vi "Autonomous Independent.vi"() -> ()   [LabVIEW 2016]
doc: "This VI is called when autonomous begins, and will automatically be terminated when autonomous ends. You can carry out timed or sensor driven robot movement independently without needing to return to the caller."
uses:
  <vilib>/Rock Robotics/WPI/Utilities/WPI_GetSetVariantRefNum.vi
  <vilib>/Rock Robotics/Network Tables/NT Write Numeric Array.vi
  Robot Global Data.vi
  <vilib>/Rock Robotics/WPI/RobotDrive/WPI_RobotDriveArcadeDrive_Standard(NoSaturation).vi
panel:
  in  "Drive to target":bool=TRUE
  in  "Auto Routine":enum16{"PID Angle Testing", "Find Target"}(ring)=enum."Find Target"
  # "Be sure to right-click and choose Data Operations>>Make Current Value default if you want to save the array values with the VI"
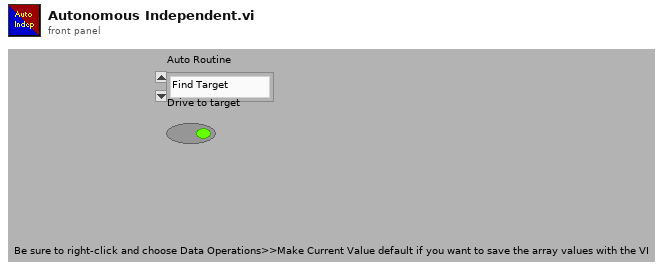
[diagram p1: front panel]
types:
  T1 = typedef "WPI_JoystickDevRef.ctl" = cluster{"Device":T2}
  T2 = typedef "WPI_JoystickDeviceEnum.ctl" = enum16{"USB 0", "USB 1", "USB 2", "USB 3", "USB 4", "USB 5"}
  T3 = typedef "WPI_RobotDriveDevRef.ctl" = cluster{"DevStatus":errorcluster, "Motors[]":T4[], "Square Inputs":bool, "Max Output":dbl}
  T4 = typedef "WPI_MotorControlDeviceRef.ctl" = cluster{"DeviceStatus":errorcluster, "Type":T5, "PWM":cluster{"PWM Channel":T6, "DeadBand":T7}, "CAN":cluster{"Device Number":u8, "SetOutput VI Ref":variant, "GetOutput VI Ref":variant, "Enable VI Ref":variant, "Disable VI Ref":variant, "Data":variant}, "Invert":bool}
  T5 = typedef "WPI_MotorControlType.ctl" = enum16{"PWM", "CAN"}
  T6 = typedef "FPGA_DIOPWMChannel.ctl" = enum8{"PWM 0", "PWM 1", "PWM 2", "PWM 3", "PWM 4", "PWM 5", "PWM 6", "PWM 7", "PWM 8", "PWM 9", "PWM MXP 0", "PWM MXP 1", "PWM MXP 2", "PWM MXP 3", "PWM MXP 4", "PWM MXP 5", "PWM MXP 6", "PWM MXP 7", "PWM MXP 8", "PWM MXP 9", "Invalid"}
  T7 = typedef "WPI_PWMDeadband.ctl" = cluster{"Name":string, "maxPositivePwm":i32, "minPositivePwm":i32, "centerPwm":i32, "maxNegativePwm":i32, "minNegativePwm":i32, "angularRange":u16}
  T8 = cluster{"Target?":bool, "Angle":dbl, "Distance":dbl}
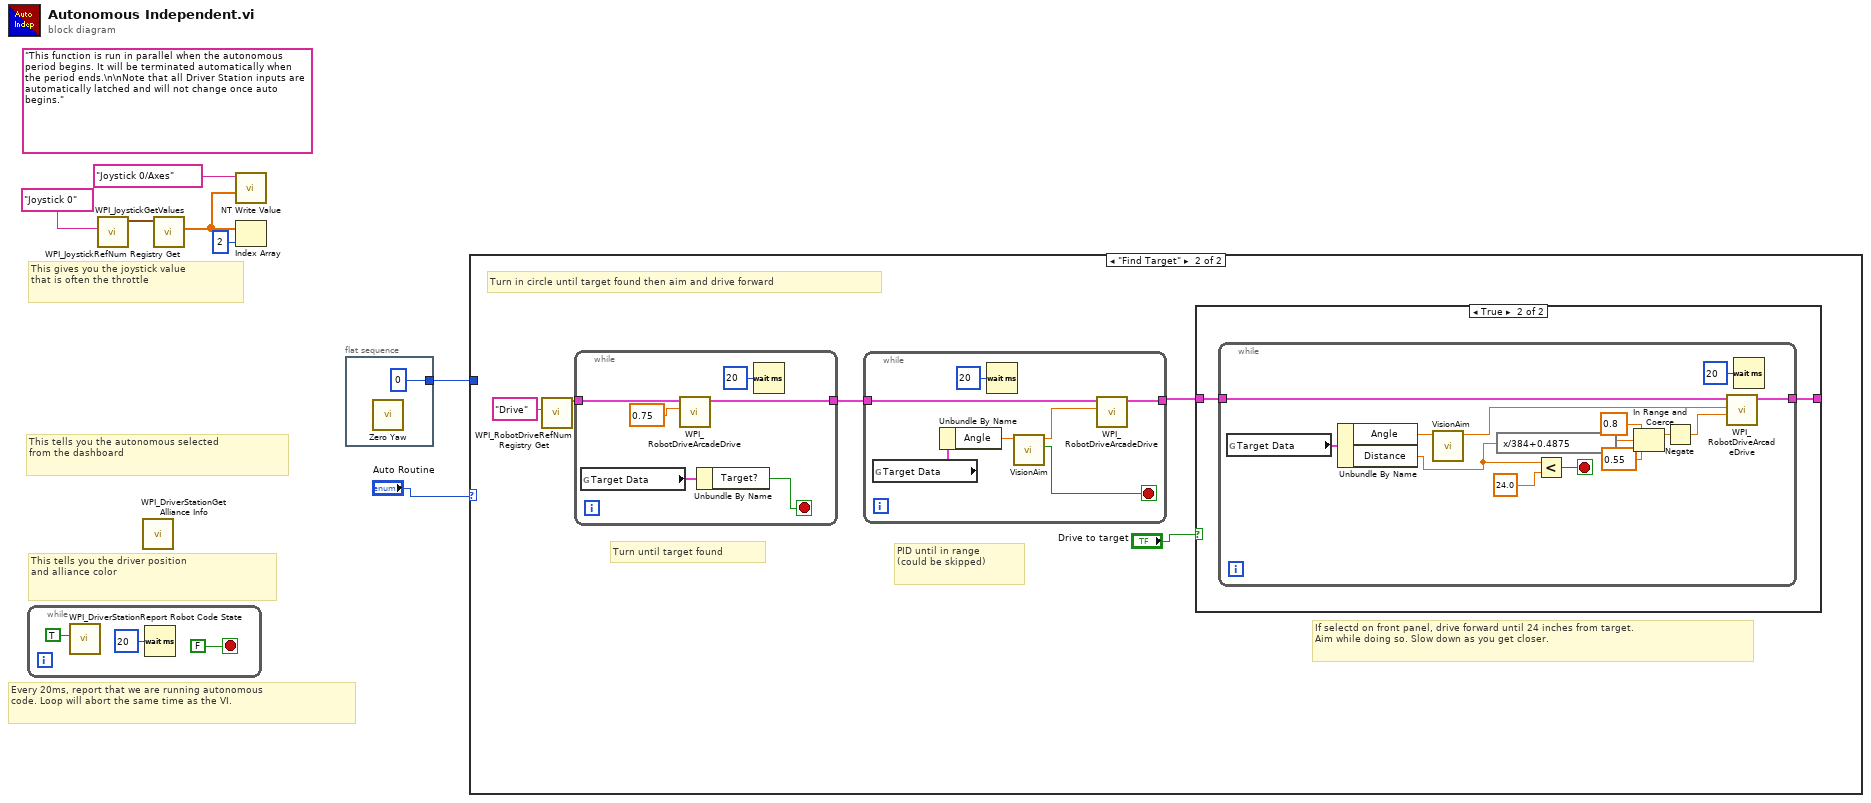
[diagram p0: block diagram]
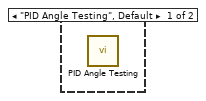
[diagram p2: hidden frame]
diagram:
  (unwired) "This function is run in parallel when the autonomous period begins. It will be terminated automatically when the period ends.\n\nNote that all Driver Station inputs are automatically latched and will not change once auto begins."
  # "This tells you the autonomous selected\nfrom the dashboard"
  # "Every 20ms, report that we are running autonomous\ncode. Loop will abort the same time as the VI."
  # "This gives you the joystick value\nthat is often the throttle"
  # "This tells you the driver position\nand alliance color"
  n1 = while {
    stop <- FALSE stop-if-true
    n2 = call <vilib>:"WPI_DriverStationReport Robot Code State.vi"("Autonomous"=TRUE) -> ()  [unwired: 10 in, 1 out]
    n3 = Wait (ms)(milliseconds to wait=u32 20) -> ()  [unwired: 1 out]
  }
  n4 = call <vilib>:"WPI_JoystickRefNum Registry Get.vi"("refnum name"="Joystick 0") -> ("JoystickDevRef"=w6:T1)  [unwired: 1 in, 9 out]
  n5 = call <vilib>:"WPI_DriverStationGet Alliance Info.vi"() -> ()  [unwired: 12 out]
  n6 = call <vilib>:"WPI_JoystickGetValues.vi"("JoystickDevRef"=w6) -> ("Axes"=w4:dbl[])  [unwired: 6 in, 4 out]
  n7 = call-poly <vilib>:"NT Write Value.vi"("Numeric Array"=w4, "Name"="Joystick 0/Axes") -> ()  [unwired: 9 in, 1 out]
  n8 = Index Array(array=w4, index=2) -> ()  [unwired: 1 out]
  n9 = flat-sequence {
    tunnel: [u32 0 ("milliseconds to wait")] -> w1
    frame #0 {
      n10 = call <vilib>:"Zero Yaw.vi"() -> ()  [unwired: 12 in]
    }
  }
  n11 = case shown="\"Find Target\"" "Auto Routine" {
    tunnel: w1 -> [_ _]
    frame "PID Angle Testing", Default {
      n12 = call "PID Angle Testing.vi"() -> ()  [unwired: 12 in]
    }
    frame "Find Target" {
      # "If selectd on front panel, drive forward until 24 inches from target.\nAim while doing so. Slow down as you get closer."
      # "PID until in range\n(could be skipped)"
      # "Turn until target found"
      # "Turn in circle until target found then aim and drive forward"
      n13 = call <vilib>:"WPI_RobotDriveRefNum Registry Get.vi"("refnum name"="Drive") -> ("RobotDriveDevRef"=w15:T3)  [unwired: 9 in, 1 out]
      n14 = while {
        tunnel: w15 -> [w46]
        tunnel: [w44] -> w14
        stop <- w41 stop-if-true
        n15 = global read "Robot Global Data.vi" "Target Data"() -> (w42:T8)
        n16 = call-poly <vilib>:"WPI_RobotDriveArcadeDrive.vi"("X axis value"=0.75, "RobotDriveDevRef"=w46) -> ("RobotDriveDevRef"=w44:T3)  [unwired: 7 in, 2 out]
        n17 = Unbundle By Name(w42) -> ("Target?"=w41:bool)
        n18 = Wait (ms)(milliseconds to wait=u32 20) -> ()  [unwired: 1 out]
      }
      n19 = while {
        tunnel: w14 -> [w40]
        tunnel: [w36] -> w12
        stop <- w38 stop-if-true
        n20 = global read "Robot Global Data.vi" "Target Data"() -> (w35:T8)
        n21 = Unbundle By Name(w35) -> ("Angle"=w34:dbl)
        n22 = Wait (ms)(milliseconds to wait=u32 20) -> ()  [unwired: 1 out]
        n23 = call "VisionAim.vi"("Angle"=w34) -> ("In Range"=w38:bool, "Turn Amount"=w39:dbl)  [unwired: 9 in]
        n24 = call-poly <vilib>:"WPI_RobotDriveArcadeDrive.vi"("X axis value"=w39, "RobotDriveDevRef"=w40) -> ("RobotDriveDevRef"=w36:T3)  [unwired: 7 in, 2 out]
      }
      n25 = case shown="True" "Drive to target" {
        tunnel: w12 -> [w17 w19]
        tunnel: [w17 w18] -> _
        frame False {
        }
        frame True {
          n26 = while {
            tunnel: w19 -> [w32]
            tunnel: [w31] -> w18
            stop <- w29 stop-if-true
            n27 = global read "Robot Global Data.vi" "Target Data"() -> (w22:T8)
            n28 = Unbundle By Name(w22) -> ("Angle"=w21:dbl, "Distance"=w20:dbl)
            n29 = call "VisionAim.vi"("Angle"=w21) -> ("Turn Amount"=w33:dbl)  [unwired: 9 in, 1 out]
            n30 = expression code="x/384+0.4875"(w20) -> (w27:dbl)
            n31 = Less?(x=w20, y=24.0) -> (x < y?=w29:bool)
            n32 = In Range and Coerce(upper limit=0.8, x=w27, lower limit=0.55) -> (coerced(x)=w24:dbl)  [unwired: 1 out]
            n33 = Negate(x=w24) -> (-x=w23:dbl)
            n34 = call-poly <vilib>:"WPI_RobotDriveArcadeDrive.vi"("Y axis value"=w23, "X axis value"=w33, "RobotDriveDevRef"=w32) -> ("RobotDriveDevRef"=w31:T3)  [unwired: 6 in, 2 out]
            n35 = Wait (ms)(milliseconds to wait=u32 20) -> ()  [unwired: 1 out]
          }
        }
      }
    }
  }
